vi "B29xx_auto_ohms.vi"(6 "Resistance Auto Range (T: Enable)":bool=TRUE, 7 "Enable Remote Sensing (4-wire)":bool=TRUE, 11 "SMU VISA name":refnum<visa-resource-name>="GPIB1::29::INSTR") -> (0 "Error Out":errorcluster, 2 "Measured Resistance (Ohms)":dbl format="%#_6p")   [LabVIEW 2017]
panel:
  in  "Resistance Range Lower Limit (2 Ohm)":dbl=2.0 format="%#_6p"
  in  "Resistance Range Upper Limit (2E+8 Ohm)":dbl=200000000.0 format="%#_6p"
  in  "Resistance NPLC (0.1)":dbl=0.1
  in  "Resistance Range (2 Ohm)":dbl=2.0
  in  "Error In":errorcluster
  # "Keysight B29xx - Auto Resistance Measurement  (Remote Sensing)"
  # "If Auto Range Disabled use Manual Range.."
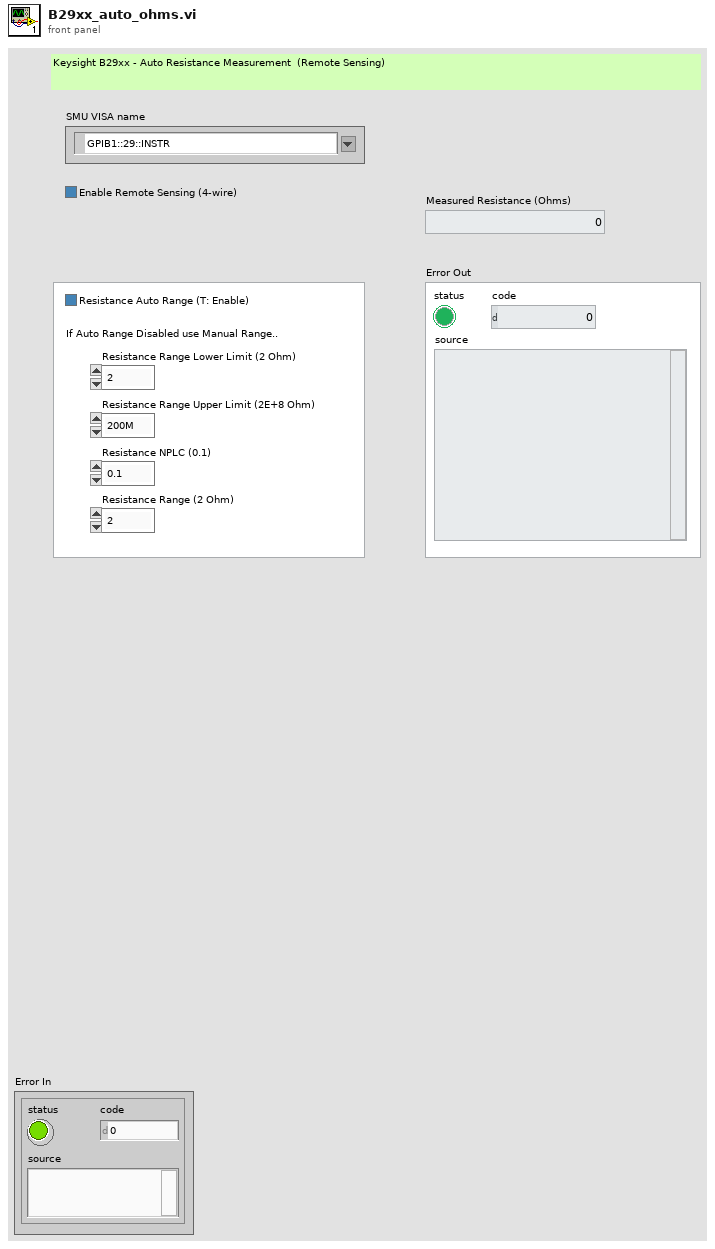
[diagram p1: front panel]
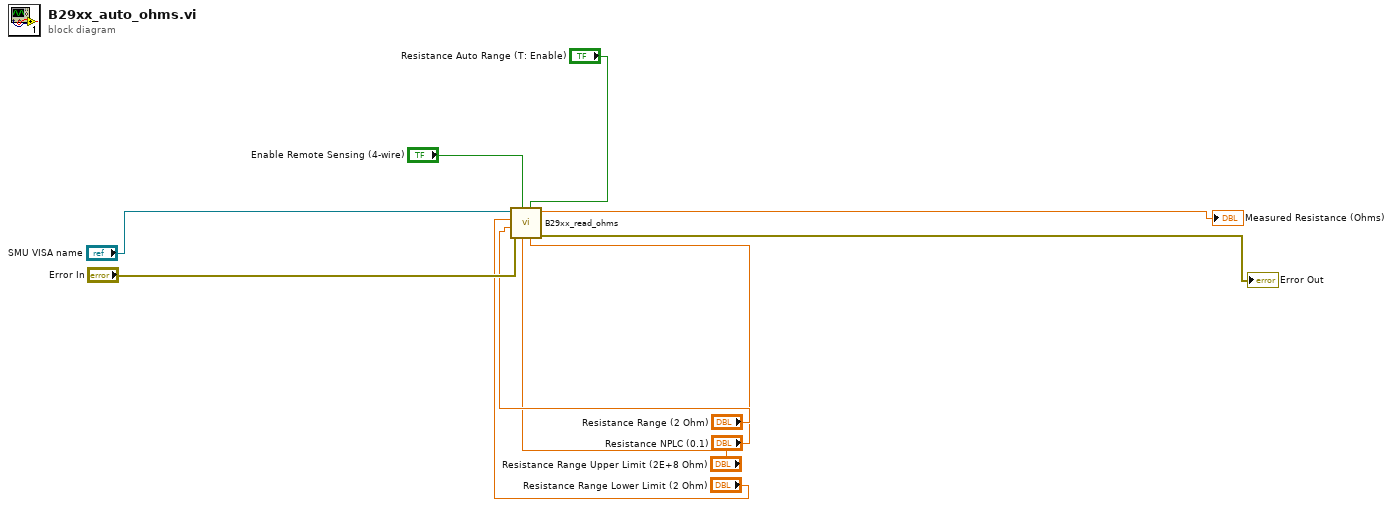
[diagram p0: block diagram]
diagram:
  n1 = call "B29xx_read_ohms.vi"("Resistance NPLC (0.1)"="Resistance NPLC (0.1)", "Resistance Auto Range (T: Enable)"="Resistance Auto Range (T: Enable)", "Resistance Range Upper Limit (2E+8 Ohm)"="Resistance Range Upper Limit (2E+8 Ohm)", "Enable Remote Sensing (4-wire)"="Enable Remote Sensing (4-wire)", "error in (no error)"="Error In", "Resistance Range (2 Ohm)"="Resistance Range (2 Ohm)", "Resistance Range Lower Limit (2 Ohm)"="Resistance Range Lower Limit (2 Ohm)", "VISA Refnum in"="SMU VISA name") -> ("error out"=→"Error Out":errorcluster, "Measurement Result"=→"Measured Resistance (Ohms)":dbl)  [unwired: 2 in]
